vi "Process data - Overview.vi"() -> ()   [LabVIEW 2021]
uses:
  <vilib>/Utility/miscctls.llb/LV3DPointTypeDef.ctl
  <vilib>/Platform/TimedLoop/XDataNode/timing_clust.ctl
  <vilib>/Platform/TimedLoop/XDataNode/nitl_modes.ctl
  <vilib>/Platform/TimedLoop/XDataNode/wakeup.ctl
  <vilib>/Analysis/baseanly.llb/Real Outer Product.vi
  <vilib>/picture/3D Picture Control/Object/Create Object (name).vi
  <vilib>/picture/3D Picture Control/Object/Create Object (drawable).vi
  <vilib>/picture/3D Picture Control/Object/Add Object (no reference).vi
  <vilib>/platform/TimedLoop/XDataNode/XDataNode.xnode
  <vilib>/Platform/TimedLoop/XDataNode/XDNodeRunTimeDep.lvlib
  <vilib>/picture/3D Picture Control/NI_3D Picture Control.lvlib
  <vilib>/gmath/NI_Gmath.lvlib
  <vilib>/Analysis/NI_AALBase.lvlib
panel:
  in  "Calibraion Length":i32=500
  in  "stop magnetometer":bool
  out "Magnetometer":refnum<vi>(3d-picture)
  out "Magnetometer corrected":refnum<vi>(3d-picture)
  in  "Calibrate":bool
  in  "Clear":bool
  in  "stop Accerelometer":bool
  in  "Enum 3":enum16{"None", "Disc", "Box", "STL"}(ring)=enum."Disc"
  out "FN RZRollY":dbl
  out "FN RYRollZ":dbl
  out "FN RXRollZ":dbl
  out "FN RZRollX":dbl
  out "FN RYRollX":dbl
  out "FN RXRollY":dbl
  in  "Camera Position":T1={"X"=1.0, "Y"=2.0, "Z"=5.0}
  out "FN ZRoll":dbl
  out "FN YRoll":dbl
  out "FN XRoll":dbl
  out "IMU":refnum<vi>(3d-picture)
  in  "DAQ Port":refnum<visa-resource-name>
  # "Other options"
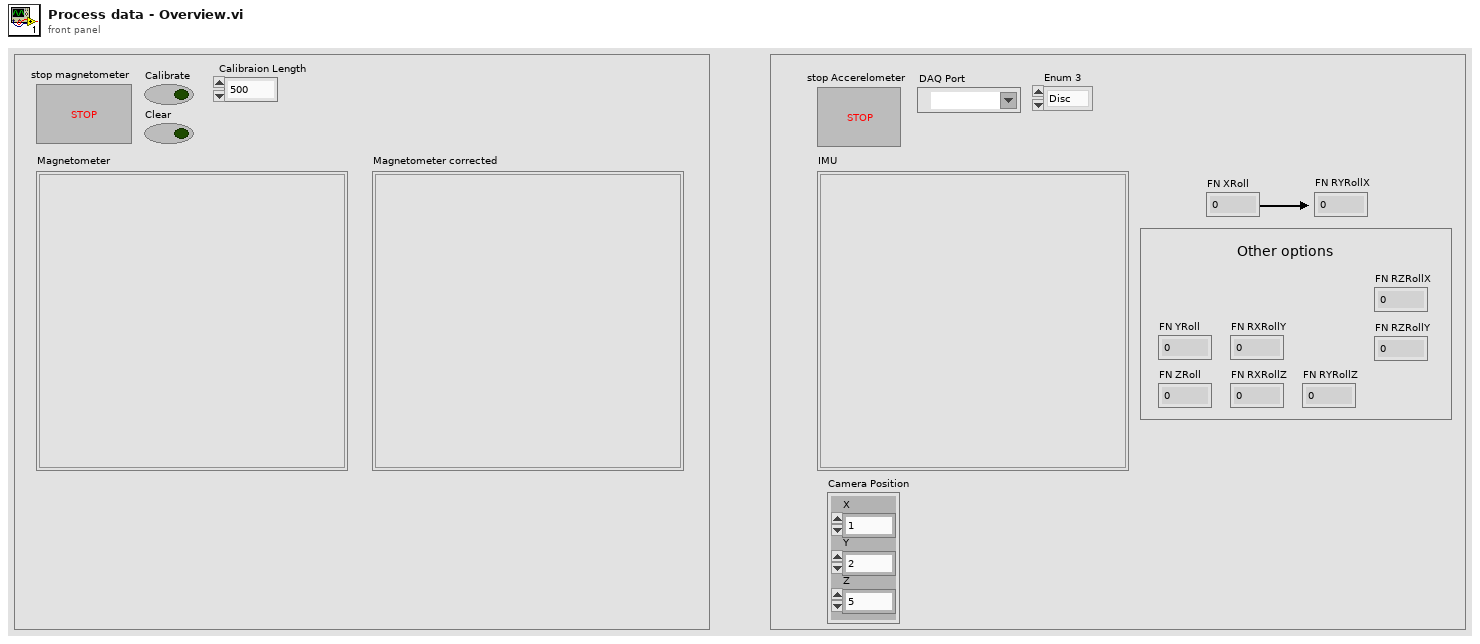
[diagram p1: front panel]
types:
  T1 = typedef "LV3DPointTypeDef.ctl" = cluster{"X":sgl, "Y":sgl, "Z":sgl}
  T2 = enum32{"Invalid", "Standard", "Closed", "Hidden", "Minimized", "Maximized"}
  T3 = cluster{"Red":sgl, "Green":sgl, "Blue":sgl, "Alpha":sgl}
  T4 = typedef "XDNodeRunTimeDep.lvlib/timing_clust.ctl" = cluster{"Expected End [f-1]":u64, "Actual End [f-1]":u64, "Finished Late? [f-1]":bool, "Expected End [i-1]":u64, "Actual End [i-1]":u64, "Finished Late? [i-1]":bool, "Expected Start [i]":u64, "Actual Start [i]":u64, "Expected Start [f]":u64, "Actual Start [f]":u64, "Source Name":string, "Structure Name":string, "Period":i64, "Deadline":i64, "Offset":i64, "Start":i64, "Priority":i32, "Timeout":i32, "Mode":T5, "Wakeup Reason":T6, "Error":errorcluster, "Source Type":string, "Secondary Source Type":string, "Global End Time":u64, "Global Start Time":u64, "Frame Duration":u64, "Iteration Duration":u64, "Assigned CPU":i32, "I/O Scan Engine Mode":u32}
  T5 = typedef "XDNodeRunTimeDep.lvlib/nitl_modes.ctl" = enum32{"No Change", "Process missed periods, maintain original phase", "Discard missed periods, maintain original phase", "Process missed periods, ignore original phase", "Discard missed periods, ignore original phase"}
  T6 = typedef "XDNodeRunTimeDep.lvlib/wakeup.ctl" = enum32{"Normal", "Aborted", "Asynchronous wakeup", "Timing source error", "Timed loop error", "Timeout"}
  T7 = cluster{"x0, y0, z0[0]":dbl, "x0, y0, z0[1]":dbl, "x0, y0, z0[2]":dbl}
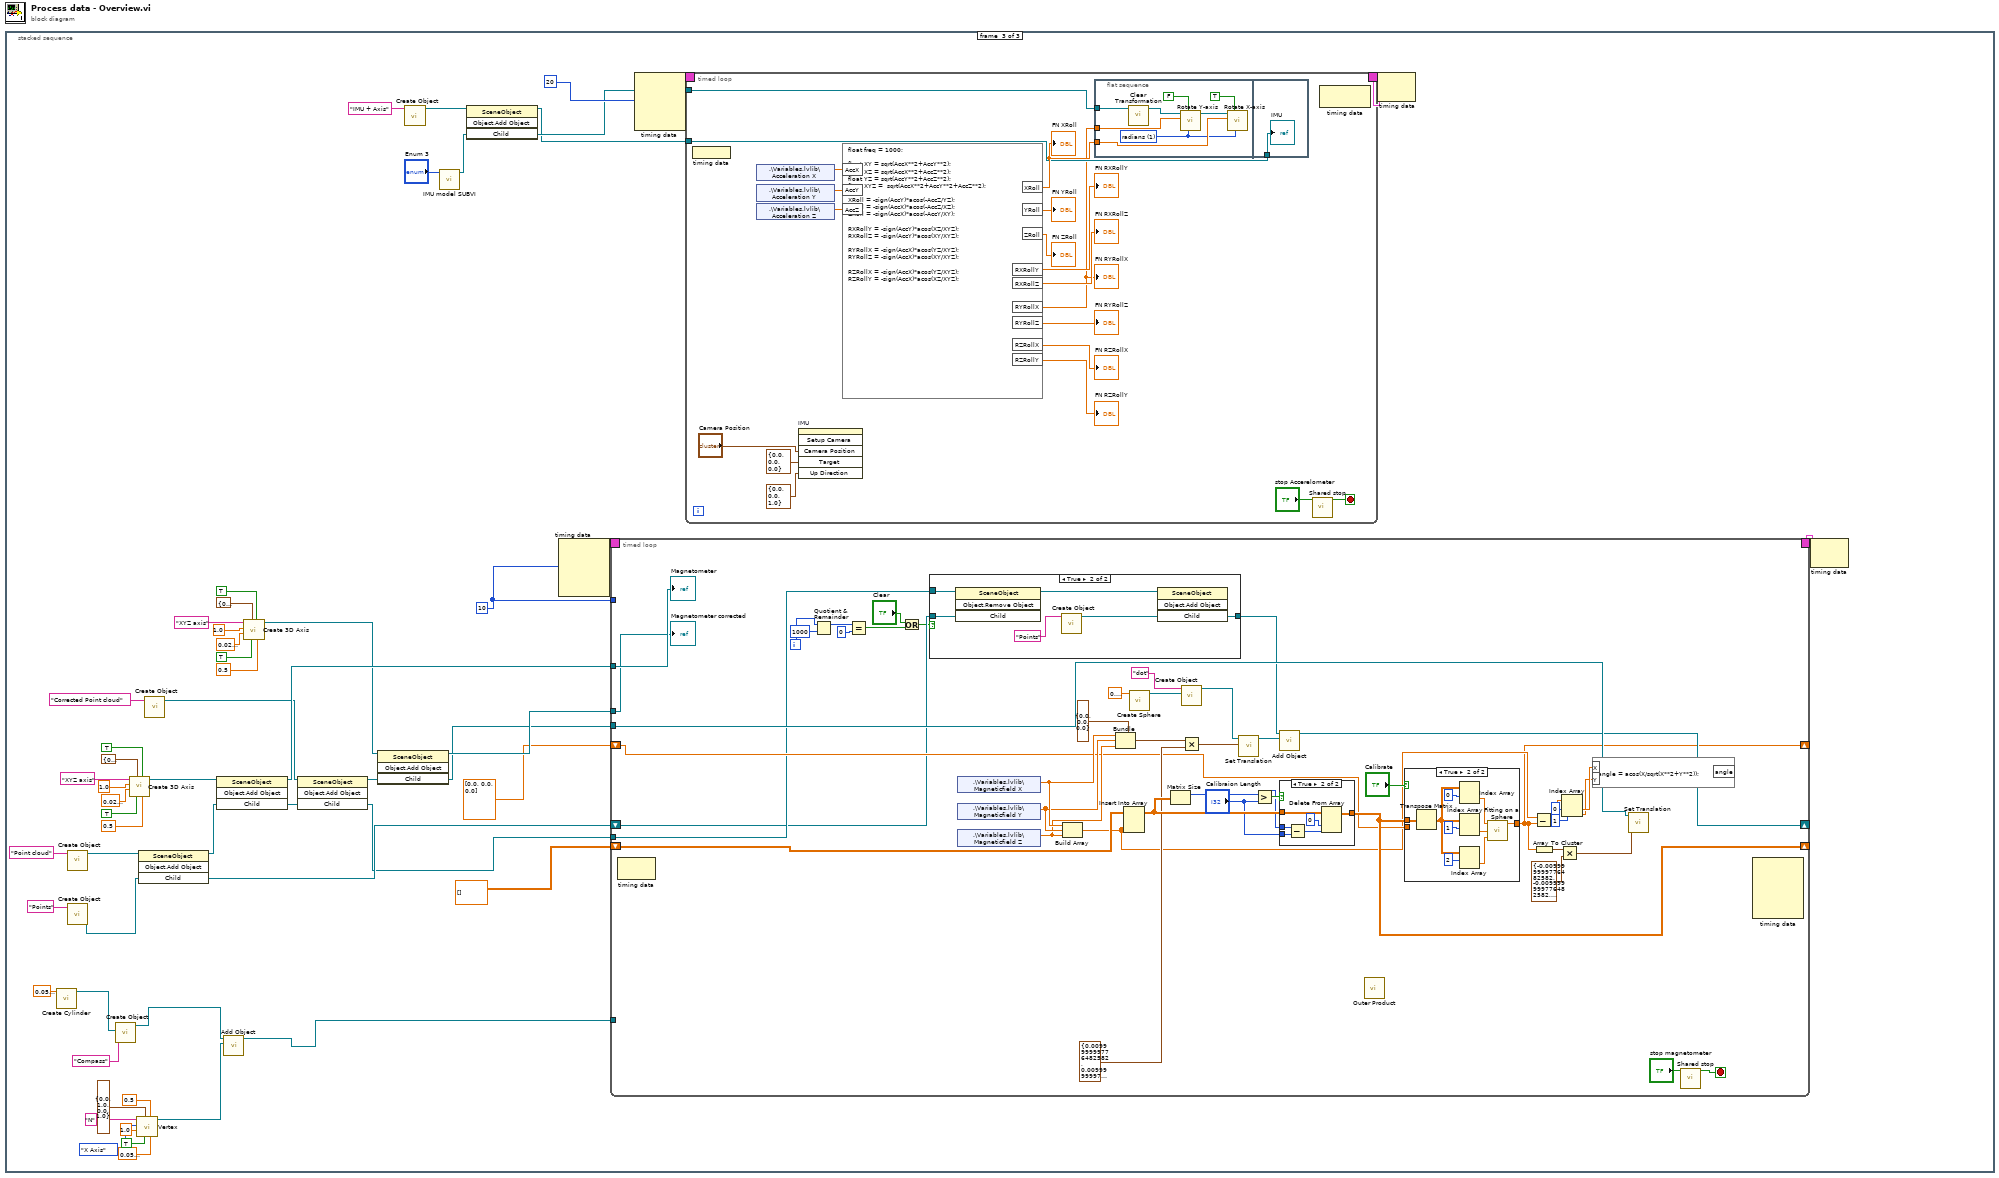
[diagram p0: block diagram]
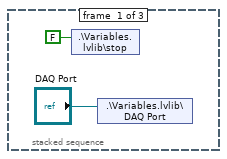
[diagram p2: hidden frame]
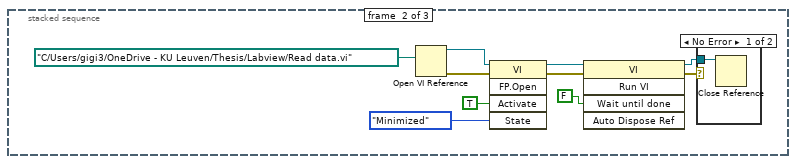
[diagram p3: hidden frame]
diagram:
  n1 = stacked-sequence {
    frame #0 {
      n2 = shared-variable ".\\Variables.lvlib\\stop"(FALSE ("stop")) -> ()  [unwired: 1 in, 1 out]
      n3 = shared-variable ".\\Variables.lvlib\\DAQ Port"("DAQ Port") -> ()  [unwired: 1 in, 1 out]
    }
    frame #1 {
      n4 = Open VI Reference(vi path=path "C:/Users/gigi3/OneDrive - KU Leuven/Thesis/Labview/Read data.vi") -> (vi reference=w12:refnum<vi>, error out=w4:errorcluster)  [unwired: 5 in]
      n5 = invoke class="VI" method="FP.Open"(reference=w12, error in=w4, "Activate"=TRUE ("Activate?"), "State"=T2."Minimized") -> (reference out=w11:refnum<vi>, error out=w5:errorcluster)  [unwired: 1 in, 3 out]
      n6 = invoke class="VI" method="Run VI"(reference=w11, error in=w5, "Wait until done"=FALSE ("Wait Until Done")) -> (reference out=w8:refnum<vi>, error out=w6:errorcluster)  [unwired: 2 in, 3 out]
      n7 = case shown="No Error" w6 {
        tunnel: w8 -> [w13 _]
        frame No Error {
          n8 = Close Reference(reference=w13) -> ()  [unwired: 1 in, 1 out]
        }
        frame Error {
        }
      }
    }
    frame #2 {
      w59 = i64 10 ("Period")
      n9 = call <vilib>:"Create Cylinder.vi"("Height"=sgl 0.05) -> ("New Cylinder Refnum"=w25:refnum<vi>)  [unwired: 9 in, 1 out]
      n10 = call-poly <vilib>:"Create Object.vi"("Name"="Point cloud") -> ("Scene:New Object"=w30:refnum<vi>)  [unwired: 9 in, 1 out]
      n11 = call-poly <vilib>:"Create Object.vi"("Name"="Points") -> ("Scene:New Object"=w32:refnum<vi>)  [unwired: 9 in, 1 out]
      n12 = call-poly <vilib>:"Create Object.vi"("Geometry"=w25, "Name"="Compass") -> ("Scene:New Object"=w16:refnum<vi>)  [unwired: 8 in, 1 out]
      n13 = call <vilib>:"Create 3D Axis.vi"("Character Size"=sgl 0.5, "Half plane?"=TRUE, "Axis label?"=TRUE, "Color"=T3 {"Red"=0.0, "Green"=1.0, "Blue"=0.0, "Alpha"=1.0}, "Radius"=sgl 0.03, "Length"=sgl 1.0, "Name"="XYZ axis") -> ("New Object Refnum"=w43:refnum<vi>)  [unwired: 3 in, 1 out]
      n14 = call "Vertex.vi"("Radius"=sgl 0.05, "Font Size"=sgl 0.5, "Vertex label?"=TRUE, "Color"=T3 {"Red"=0.0, "Green"=1.0, "Blue"=0.0, "Alpha"=1.0}, "Length"=sgl 1.0, "Enum"=enum16{"X Axis", "Y Axis", "Z Axis"}."X Axis", "Name"="N") -> ("New Object Refnum"=w15:refnum<vi>)  [unwired: 3 in, 1 out]
      n15 = invoke class="SceneObject" method="Object.Add Object"(reference=w30, "Child"=w32) -> (reference out=w31:refnum<vi>, "Child"=w29:refnum<vi>)  [unwired: 2 in, 2 out]
      n16 = call-poly <vilib>:"Create Object.vi"("Name"="Corrected Point cloud") -> ("Scene:New Object"=w39:refnum<vi>)  [unwired: 9 in, 1 out]
      n17 = invoke class="SceneObject" method="Object.Add Object"(reference=w43, "Child"=w31) -> (reference out=w42:refnum<vi>, "Child"=w34:refnum<vi>)  [unwired: 2 in, 2 out]
      n18 = call-poly <vilib>:"Add Object.vi"("New Object In"=w15, "Scene Object In"=w16) -> ("Scene Object Out"=w14:refnum<vi>)  [unwired: 8 in, 1 out]
      n19 = call <vilib>:"Create 3D Axis.vi"("Character Size"=sgl 0.5, "Half plane?"=TRUE, "Axis label?"=TRUE, "Color"=T3 {"Red"=0.0, "Green"=1.0, "Blue"=0.0, "Alpha"=1.0}, "Radius"=sgl 0.03, "Length"=sgl 1.0, "Name"="XYZ axis") -> ("New Object Refnum"=w38:refnum<vi>)  [unwired: 3 in, 1 out]
      n20 = invoke class="SceneObject" method="Object.Add Object"(reference=w39, "Child"=w34) -> (reference out=w37:refnum<vi>, "Child"=w28:refnum<vi>)  [unwired: 2 in, 2 out]
      n21 = invoke class="SceneObject" method="Object.Add Object"(reference=w38, "Child"=w37) -> (reference out=w36:refnum<vi>, "Child"=w35:refnum<vi>)  [unwired: 2 in, 2 out]
      n22 = call-poly <vilib>:"Create Object.vi"("Name"="IMU + Axis") -> ("Scene:New Object"=w62:refnum<vi>)  [unwired: 9 in, 1 out]
      n23 = call "IMU model SUBVI.vi"("Enum 3"="Enum 3") -> ("SceneObject out"=w63:refnum<vi>)  [unwired: 10 in]
      n24 = invoke class="SceneObject" method="Object.Add Object"(reference=w62, "Child"=w63) -> (reference out=w64:refnum<vi>, "Child"=w65:refnum<vi>)  [unwired: 2 in, 2 out]
      n25 = node-c288(w59) -> (w61:T4)  [unwired: 3 in]
      n26 = timed-loop {
        timing: w61 -> [_]
        timing-out: [_] -> w60
        tunnel: w59 -> [_]
        shift-right: [w112] -> _
        shift-left: dbl[][] [] -> [w115]
        tunnel: w42 -> [w99]
        tunnel: w36 -> [w98]
        tunnel: w35 -> [w97]
        shift-right: [w78] -> _
        shift-left: dbl[] [0.0, 0.0, 0.0] ("x0, y0, z0") -> [w95]
        tunnel: w28 -> [w93]
        shift-right: [w91] -> _
        shift-left: w29 -> [w90]
        tunnel: w14 -> [_]
        i -> [w87]
        stop <- w83 stop-if-true
        n27 = node-c288() -> ()  [unwired: 1 in, 1 out]
        n28 = Quotient & Remainder(x=w87, y=1000) -> (x-y*floor(x/y)=w84:i32)  [unwired: 1 out]
        n29 = Equal?(x=w84, y=0) -> (x = y?=w86:bool)
        n30 = Or(x="Clear", y=w86) -> (x .or. y?=w89:bool)
        n31 = case shown="True" w89 {
          tunnel: w93 -> [_ w123]
          tunnel: [w117 w118] -> w92
          tunnel: w90 -> [w117 w119]
          frame False {
          }
          frame True {
            n32 = invoke class="SceneObject" method="Object.Remove Object"(reference=w123, "Child"=w119) -> (reference out=w121:refnum<vi>)  [unwired: 2 in, 3 out]
            n33 = call-poly <vilib>:"Create Object.vi"("Name"="Points") -> ("Scene:New Object"=w120:refnum<vi>)  [unwired: 9 in, 1 out]
            n34 = invoke class="SceneObject" method="Object.Add Object"(reference=w121, "Child"=w120) -> ("Child"=w118:refnum<vi>)  [unwired: 2 in, 3 out]
          }
        }
        n35 = shared-variable ".\\Variables.lvlib\\Magneticfield X"() -> (w103:dbl)  [unwired: 1 in, 1 out]
        n36 = shared-variable ".\\Variables.lvlib\\Magneticfield Y"() -> (w102:dbl)  [unwired: 1 in, 1 out]
        n37 = shared-variable ".\\Variables.lvlib\\Magneticfield Z"() -> (w101:dbl)  [unwired: 1 in, 1 out]
        n38 = Build Array(w103, w102, w101) -> (w82:dbl[])
        n39 = Bundle(cluster=cluster{"X":sgl, "Y":sgl, "Z":sgl} {"X"=0.0, "Y"=0.0, "Z"=0.0} ("Translation"), "X"=w103, "Y"=w102, "Z"=w101) -> (w106:cluster{"X":sgl, "Y":sgl, "Z":sgl})
        n40 = Insert Into Array(array=w115, new element=w82) -> (w114:dbl[][])  [unwired: 2 in]
        n41 = call <vilib>:"Create Sphere.vi"("Radius"=sgl 0.1) -> ("New Sphere Refnum"=w110:refnum<vi>)  [unwired: 9 in, 1 out]
        n42 = Matrix Size(0:w114) -> (1:w72:i32)  [unwired: 1 out]
        n43 = call-poly <vilib>:"Create Object.vi"("Geometry"=w110, "Name"="dot") -> ("Scene:New Object"=w108:refnum<vi>)  [unwired: 8 in, 1 out]
        n44 = Multiply(x=w106, y=cluster{"X":sgl, "Y":sgl, "Z":sgl} {"X"=0.01, "Y"=0.01, "Z"=0.01}) -> (x*y=w104:cluster{"X":sgl, "Y":sgl, "Z":sgl})
        n45 = call <vilib>:"Set Translation.vi"("Translation"=w104, "Scene Object"=w108) -> ("Translated Object"=w107:refnum<vi>)  [unwired: 8 in, 1 out]
        n46 = Greater?(x=w72, y="Calibraion Length") -> (0:w113:bool)
        n47 = call-poly <vilib>:"Add Object.vi"("New Object In"=w107, "Scene Object In"=w92) -> ("Scene Object Out"=w91:refnum<vi>)  [unwired: 8 in, 1 out]
        n48 = case shown="True" w113 {
          tunnel: w114 -> [w134 w140]
          tunnel: [w134 w138] -> w112
          tunnel: w72 -> [_ w136]
          tunnel: "Calibraion Length" -> [_ w135]
          frame False {
          }
          frame True {
            n49 = Subtract(x=w136, y=w135) -> (x-y=w137:i32)
            n50 = Delete From Array(array=w140, length=w137, index (row)=0) -> (array with subset deleted=w138:dbl[][])  [unwired: 1 in, 1 out]
          }
        }
        n51 = call-poly <vilib>:"Outer Product.vi"() -> ()  [unwired: 2 in, 2 out]
        n52 = case shown="True" "Calibrate" {
          tunnel: w112 -> [_ w133]
          tunnel: w95 -> [w124 _]
          tunnel: [w124 w125] -> w78
          frame False {
          }
          frame True {
            n53 = Transpose Matrix(1:w133) -> (0:w128:dbl[][])
            n54 = Index Array(array=w128, index (row)=0) -> (element=w132:dbl[])  [unwired: 1 in]
            n55 = Index Array(array=w128, index (row)=1) -> (element=w127:dbl[])  [unwired: 1 in]
            n56 = Index Array(array=w128, index (row)=2) -> (element=w126:dbl[])  [unwired: 1 in]
            n57 = call <vilib>:"Fitting on a Sphere.vi"("Z"=w126, "Y"=w127, "X"=w132) -> ("x0, y0, z0"=w125:dbl[])  [unwired: 2 out]
          }
        }
        n58 = Subtract(x=w82, y=w78) -> (x-y=w77:dbl[])
        n59 = Array To Cluster(array=w78) -> (cluster=w80:T7)
        n60 = Multiply(x=w80, y=cluster{"X":sgl, "Y":sgl, "Z":sgl} {"X"=-0.01, "Y"=-0.01, "Z"=-0.01}) -> (x*y=w79:cluster{dbl, dbl, dbl})
        n61 = Index Array(array=w77, index #1=0 ("index"), index #2=1 ("index")) -> (element #1=w74:dbl, element #2=w73:dbl)
        n62 = formula code="angle = acos(X/sqrt(X**2+Y**2));"("X"=w74, "Y"=w73) -> ()  [unwired: 1 out]
        n63 = call <vilib>:"Set Translation.vi"("Translation"=w79, "Scene Object"=w97) -> ()  [unwired: 8 in, 2 out]
        n64 = call "Shared stop.vi"("stop"="stop magnetometer") -> ("stop 2"=w83:bool)  [unwired: 10 in]
        n65 = node-c288() -> ()  [unwired: 5 in, 1 out]
        "Magnetometer" <- w99
        "Magnetometer corrected" <- w98
      }
      n66 = node-c288(i64 20 ("Period")) -> (w70:T4)  [unwired: 3 in]
      n67 = timed-loop {
        timing: w70 -> [_]
        timing-out: [_] -> w69
        tunnel: w64 -> [w150]
        tunnel: w65 -> [w151]
        stop <- w147 stop-if-true
        n68 = node-c288() -> ()  [unwired: 1 in]
        n69 = shared-variable ".\\Variables.lvlib\\Acceleration X"() -> (w162:dbl)  [unwired: 1 in, 1 out]
        n70 = shared-variable ".\\Variables.lvlib\\Acceleration Y"() -> (w161:dbl)  [unwired: 1 in, 1 out]
        n71 = shared-variable ".\\Variables.lvlib\\Acceleration Z"() -> (w160:dbl)  [unwired: 1 in, 1 out]
        n72 = invoke on="IMU" class="SceneGraphDisp (strict)" method="Setup Camera"("Camera Position"="Camera Position", "Target"=T1 {"X"=0.0, "Y"=0.0, "Z"=0.0}, "Up Direction"=T1 {"X"=0.0, "Y"=0.0, "Z"=1.0}) -> ()  [unwired: 3 in, 6 out]
        n73 = formula code="float freq = 1000;\n\nfloat XY = sqrt(AccX**2+AccY**2);\nfloat XZ = sqrt(AccX**2+AccZ**2);\nfloat YZ = sqrt(AccY**2+AccZ**2);\nfloat XYZ =  sqrt(AccX**2+AccY**2+AccZ**2);\n\nXRoll = -sign(AccY)*acos(-AccZ/YZ);\nYRoll = -sign(AccX)*acos(-AccZ/XZ);\nZRoll = -sign(AccX)*acos(-AccY/XY);\n\nRXRollY = -sign(AccY)*acos(XZ/XYZ);\nRXRollZ = -sign(AccY)*acos(XY/XYZ);\n\nRYRollX = -sign(AccX)*acos(YZ/XYZ);\nRYRollZ = -sign(AccX)*acos(XY/XYZ);\n\nRZRollX = -sign(AccX)*acos(YZ/XYZ);\nRZRollY = -sign(AccX)*acos(XZ/XYZ);"("AccX"=w162, "AccY"=w161, "AccZ"=w160) -> ("XRoll"=w159:dbl, "YRoll"=→"FN YRoll":dbl, "ZRoll"=→"FN ZRoll":dbl, "RXRollY"=→"FN RXRollY":dbl, "RYRollX"=w149:dbl, "RZRollX"=→"FN RZRollX":dbl, "RXRollZ"=→"FN RXRollZ":dbl, "RYRollZ"=→"FN RYRollZ":dbl, "RZRollY"=→"FN RZRollY":dbl)
        "FN XRoll" <- w159
        "FN RYRollX" <- w149
        n74 = flat-sequence {
          tunnel: w159 -> [w173]
          tunnel: w149 -> [w171]
          tunnel: w151 -> [w168]
          tunnel: w150 -> [w174]
          frame #0 {
            w170 = u16 1 items=["degree", "radians"] ("angle unit")
            n75 = call <vilib>:"Clear Transformation.vi"("Object Refnum In"=w168) -> ("Object Refnum Out"=w167:refnum<vi>)  [unwired: 9 in, 1 out]
            n76 = call <vilib>:"Rotate Y-axis.vi"("angle unit"=w170, "Relative?"=FALSE, "angle"=w171, "Scene Object In"=w167) -> ("Scene Object Out"=w166:refnum<vi>)  [unwired: 6 in, 1 out]
            n77 = call <vilib>:"Rotate X-axis.vi"("angle unit"=w170, "Relative?"=TRUE, "angle"=w173, "Scene Object In"=w166) -> ()  [unwired: 6 in, 2 out]
          }
          frame #1 {
            "IMU" <- w174
          }
        }
        n78 = call "Shared stop.vi"("stop"="stop Accerelometer") -> ("stop 2"=w147:bool)  [unwired: 10 in]
        n79 = node-c288() -> ()  [unwired: 1 in, 1 out]
      }
      n80 = node-c288(w69) -> ()  [unwired: 1 out]
      n81 = node-c288(w60) -> ()  [unwired: 1 out]
    }
  }
